vi "ArmExecute.vi"   [LabVIEW 2020]
doc: "Execute Arm VI's\nInputs:\n\nOutputs:"
uses:
  ArmGamePiecePreset.ctl
  <vilib>/Rock Robotics/WPI/ThirdParty/JAS_Junk/TrajLib/Timer_New.vi
  ArmGlobal.vi
  <vilib>/Utility/semaphor.llb/Obtain Semaphore Reference.vi
  <vilib>/Rock Robotics/WPI/ThirdParty/JAS_Junk/TrajLib/Timer_Reset.vi
  <vilib>/Rock Robotics/WPI/ThirdParty/JAS_Junk/TrajLib/Timer_Start.vi
  <vilib>/Rock Robotics/WPI/ThirdParty/JAS_Junk/TrajLib/Timer_HasPeriodPassedOnce.vi
  <vilib>/Rock Robotics/Network Tables/NT Write Boolean.vi
  <vilib>/Rock Robotics/WPI/ThirdParty/JAS_Junk/TrajLib/Trajectory_Library.lvlib
  <vilib>/Rock Robotics/WPI/ThirdParty/PhotonVisionLib/PhotonVisionLib.lvlib
types:
  T1 = typedef "ArmGamePiecePreset.ctl" = enum16{"Cube", "Cone"}
  T2 = typedef "WPI_MotorControlDeviceRef.ctl" = cluster{"DeviceStatus":errorcluster, "Type":T3, "PWM":cluster{"PWM Channel":T4, "DeadBand":T5}, "CAN":cluster{"Device Number":u8, "SetOutput VI Ref":variant, "GetOutput VI Ref":variant, "Enable VI Ref":variant, "Disable VI Ref":variant, "Data":variant}, "Invert":bool, "DIO PWM":cluster{"PWM \"Enable\" Channel":T4, "DIOChannel":T6, "PWM Rate":dbl}}
  T3 = typedef "WPI_MotorControlType.ctl" = enum16{"PWM", "CAN", "DIO PWM"}
  T4 = typedef "FPGA_DIOPWMChannel.ctl" = enum8{"PWM 0", "PWM 1", "PWM 2", "PWM 3", "PWM 4", "PWM 5", "PWM 6", "PWM 7", "PWM 8", "PWM 9", "PWM MXP 0", "PWM MXP 1", "PWM MXP 2", "PWM MXP 3", "PWM MXP 4", "PWM MXP 5", "PWM MXP 6", "PWM MXP 7", "PWM MXP 8", "PWM MXP 9", "Invalid"}
  T5 = typedef "WPI_PWMDeadband.ctl" = cluster{"Name":string, "maxPositivePwm":i32, "minPositivePwm":i32, "centerPwm":i32, "maxNegativePwm":i32, "minNegativePwm":i32, "angularRange":u16}
  T6 = typedef "FPGA_DIOChannel.ctl" = enum8{"DIO 0", "DIO 1", "DIO 2", "DIO 3", "DIO 4", "DIO 5", "DIO 6", "DIO 7", "DIO 8", "DIO 9", "DIO MXP 0", "DIO MXP 1", "DIO MXP 2", "DIO MXP 3", "DIO MXP 4", "DIO MXP 5", "DIO MXP 6", "DIO MXP 7", "DIO MXP 8", "DIO MXP 9", "DIO MXP 10", "DIO MXP 11", "DIO MXP 12", "DIO MXP 13", "DIO MXP 14", "DIO MXP 15", "SPI Port CS1", "SPI Port CS2", "SPI Port CS3", "SPI Port MISO", "SPI Port MOSI", "Invalid"}
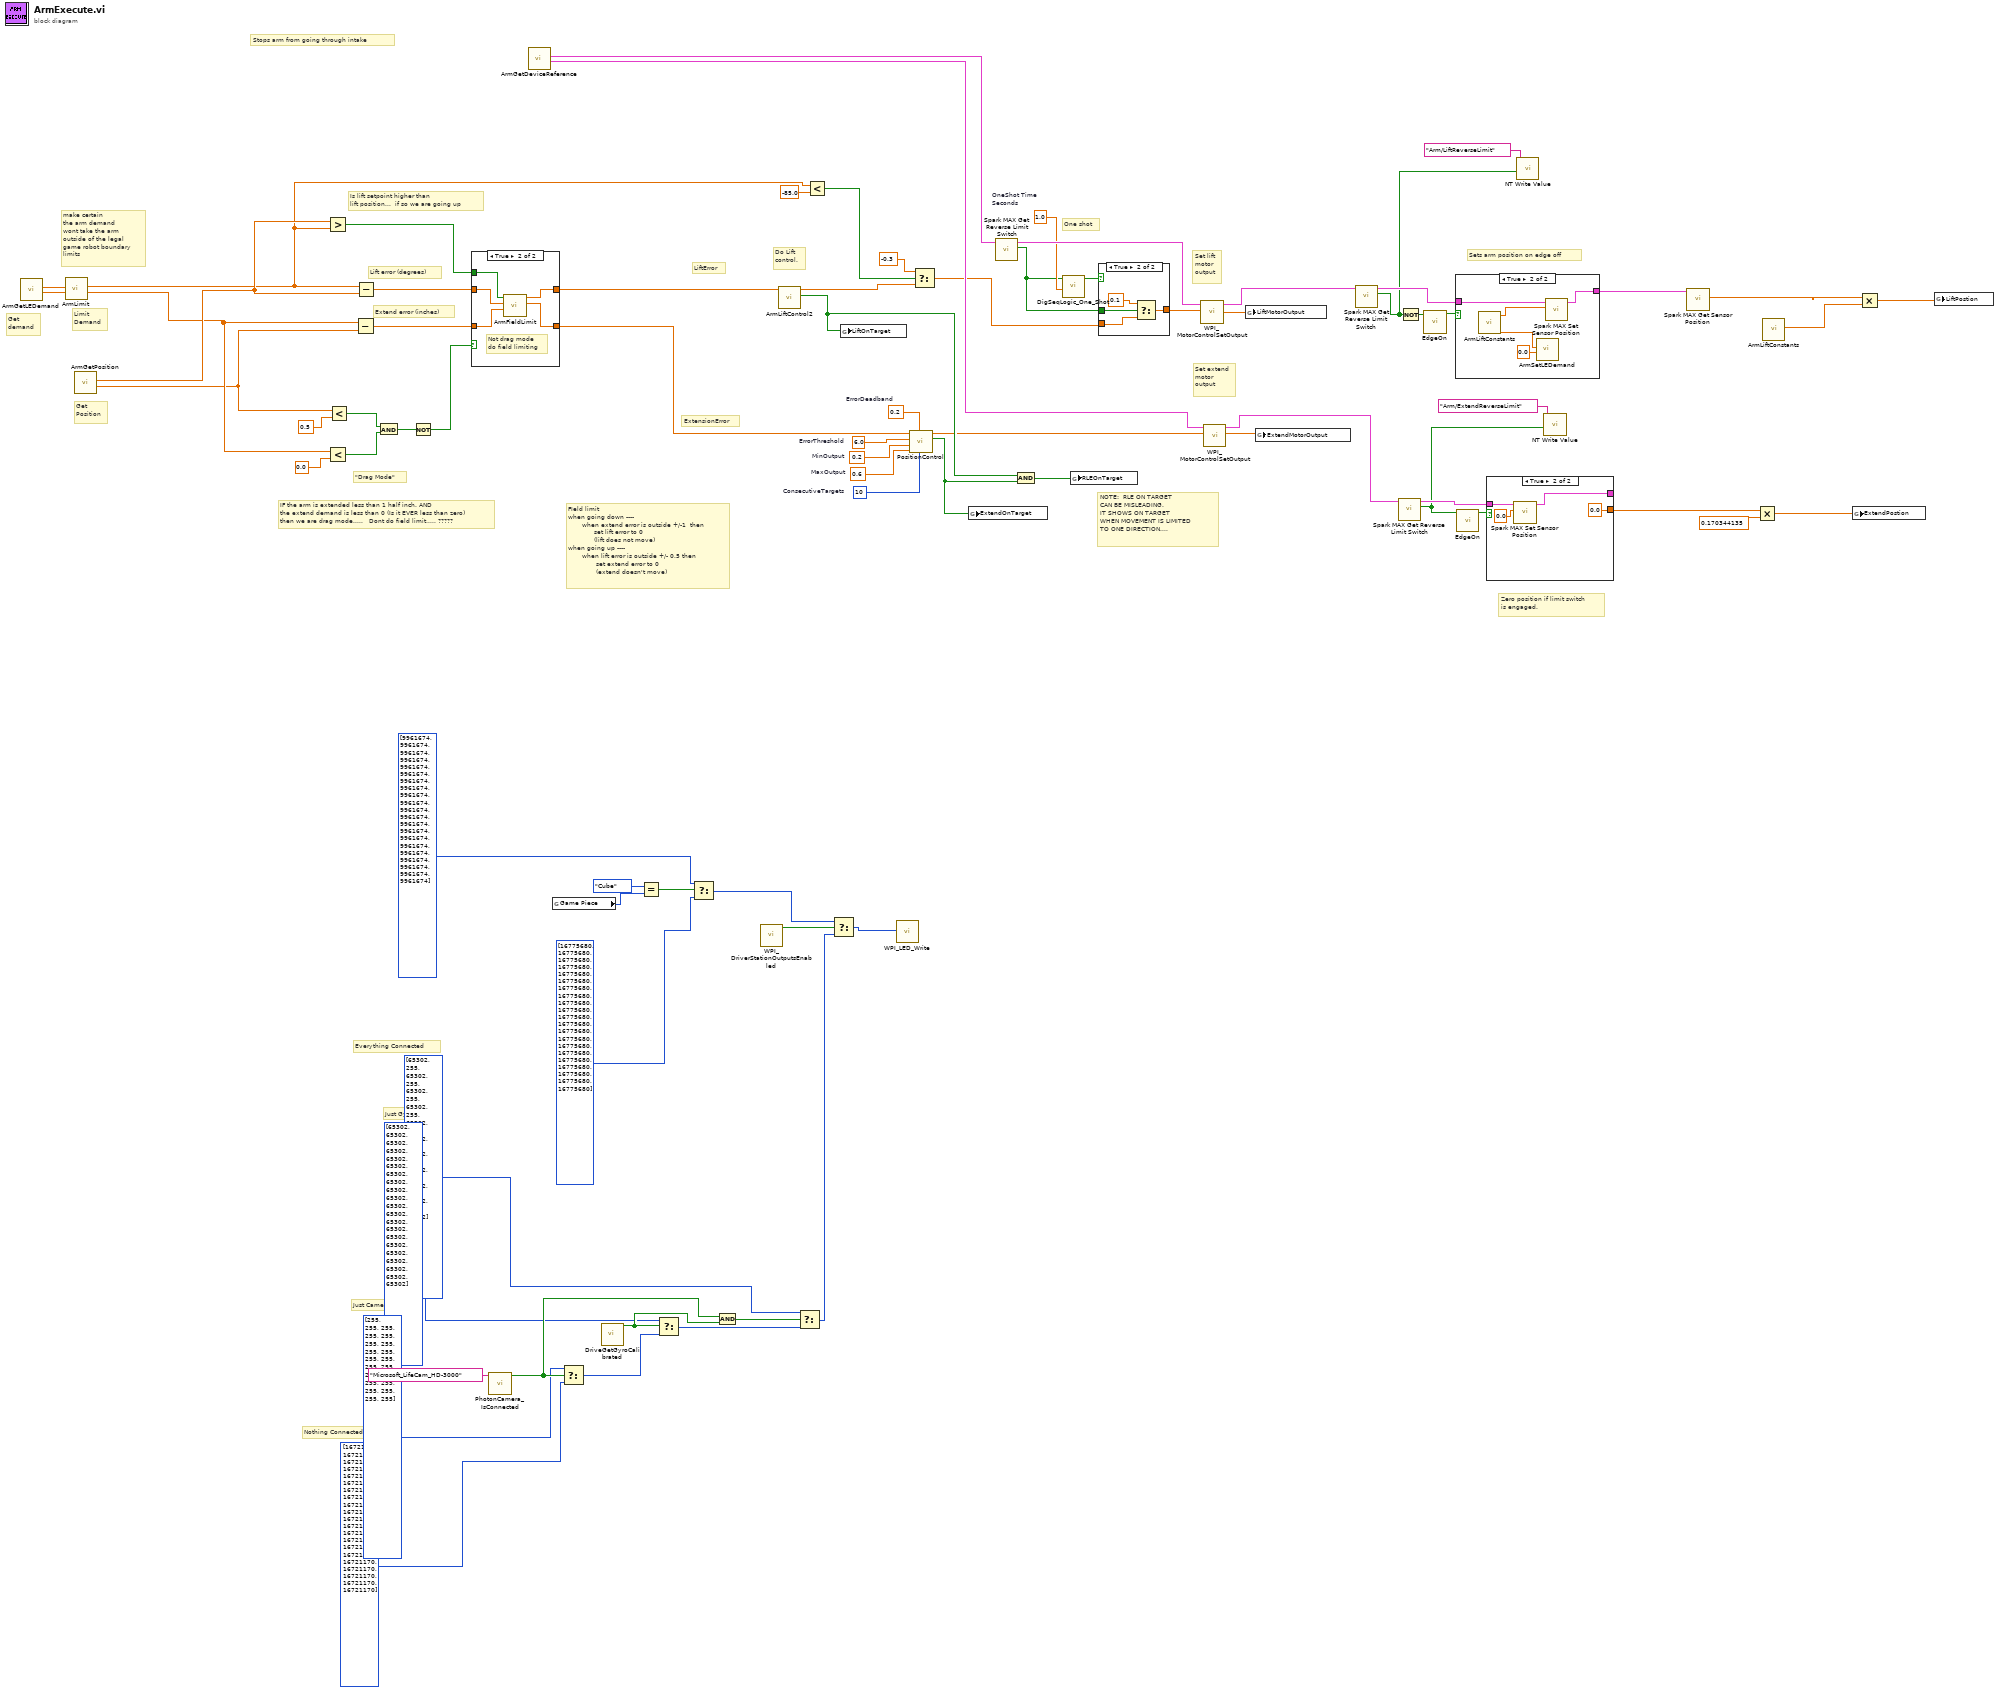
[diagram p0: block diagram]
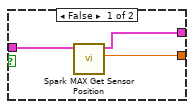
[diagram p5: hidden frame]
diagram:
  w25 = 1.0  # OneShot Time Seconds
  w70 = 10  # ConsecutiveTargets
  w71 = 0.6  # MaxOutput
  w72 = 0.2  # MinOutput
  w73 = 6.0  # ErrorThreshold
  w74 = 0.2  # ErrorDeadband
  # "Zero position if limit switch\nis engaged."
  # "Set extend\nmotor\noutput"
  # "Set lift\nmotor\noutput"
  # "Do Lift\ncontrol."
  # "Extend error (inches)"
  # "Lift error (degrees)"
  # "NOTE:  RLE ON TARGET\nCAN BE MISLEADING.\nIT SHOWS ON TARGET\nWHEN MOVEMENT IS LIMITED \nTO ONE DIRECTION...."
  # "Get\nPosition"
  # "Limit\nDemand"
  # "Get\ndemand"
  # "make certain\nthe arm demand\nwont take the arm\noutside of the legal\ngame robot boundary\nlimits"
  # "FIeld limit\nwhen going down ----\n       when extend error is outside +/-1  then\n             set lift error to 0\n             (lift does not move)\nwhen going up ----\n       when lift error is outside +/- 0.5 then\n              set extend error to 0\n              (extend doesn't move)"
  # "IF the arm is extended less than 1 half inch. AND\nthe extend demand is less than 0 (Is it EVER less than zero)\nthen we are drag mode.....   Dont do field limit..... ?????"
  # "Is lift setpoint higher than\nlift position...  if so we are going up"
  # "Everything Connected"
  # "Just Gyro"
  # "Just Camera"
  # "Nothing Connected"
  # "One shot"
  # "Sets arm position on edge off"
  # "\"Drag Mode\""
  # "Stops arm from going through intake"
  # "ExtensionError"
  # "LiftError"
  n1 = call "ArmGetLEDemand.vi"() -> ("ExtendPositonDemand(in)"=w62:dbl, "LiftPositionDemand(d)"=w63:dbl)  [unwired: 10 in]
  n2 = call "ArmLimit.vi"("Extend"=w62, "Lift"=w63) -> ("Extend"=w31:dbl, "Lift"=w38:dbl)  [unwired: 8 in]
  n3 = call "ArmGetPosition.vi"() -> ("ExtendPostion"=w28:dbl, "LiftPostion"=w51:dbl)  [unwired: 10 in]
  n4 = Greater?(x=w51, y=w38) -> (0:w54:bool)
  n5 = Less?(x=w31, y=0.0) -> (x < y?=w29:bool)
  n6 = Less?(x=w28, y=0.5) -> (x < y?=w30:bool)
  n7 = Subtract(x=w31, y=w28) -> (x-y=w55:dbl)
  n8 = Subtract(x=w38, y=w51) -> (x-y=w50:dbl)
  n9 = And(x=w30, y=w29) -> (x .and. y?=w26:bool)
  n10 = Not(x=w26) -> (.not. x?=w22:bool)
  n11 = case shown="True" w22 {
    tunnel: w55 -> [w78 w84]
    tunnel: w50 -> [w79 w83]
    tunnel: w54 -> [_ w82]
    tunnel: [w79 w81] -> w53
    tunnel: [w78 w80] -> w52
    frame False {
    }
    frame True {
      # "Not drag mode\ndo field limiting"
      n12 = call "ArmFieldLimit.vi"("Extend Error"=w84, "Lift Error"=w83, "Going Down?"=w82) -> ("Extend Error"=w80:dbl, "Lift Error"=w81:dbl)  [unwired: 7 in]
    }
  }
  n13 = call <vilib>:"PhotonCamera_IsConnected.vi"("CameraName"="Microsoft_LifeCam_HD-3000") -> ("IsConnected"=w6:bool)  [unwired: 9 in, 1 out]
  n14 = call "ArmGetDeviceReference.vi"() -> ("armExtend"=w77:T2, "armLift"=w42:T2)  [unwired: 10 in]
  n15 = global read "ArmGlobal.vi" "Game Piece"() -> (w21:T1)
  n16 = Select(t=u32[] [255, 255, 255, 255, 255, 255, 255, 255, 255, 255, 255, 255, 255, 255, 255, 255, 255, 255, 255, 255, 255] ("Color Array"), s=w6, f=u32[] [16721170, 16721170, 16721170, 16721170, 16721170, 16721170, 16721170, 16721170, 16721170, 16721170, 16721170, 16721170, 16721170, 16721170, 16721170, 16721170, 16721170, 16721170, 16721170, 16721170, 16721170] ("Color Array")) -> (s? t:f=w11:u32[])
  n17 = call "DriveGetGyroCalibrated.vi"() -> ("GryoCalibrated"=w7:bool)  [unwired: 11 in]
  n18 = Equal?(x=ArmGamePiecePreset."Cube", y=w21) -> (x = y?=w19:bool)
  n19 = Select(t=u32[] [65302, 65302, 65302, 65302, 65302, 65302, 65302, 65302, 65302, 65302, 65302, 65302, 65302, 65302, 65302, 65302, 65302, 65302, 65302, 65302, 65302] ("Color Array"), s=w7, f=w11) -> (s? t:f=w9:u32[])
  n20 = Select(t=u32[] [9961674, 9961674, 9961674, 9961674, 9961674, 9961674, 9961674, 9961674, 9961674, 9961674, 9961674, 9961674, 9961674, 9961674, 9961674, 9961674, 9961674, 9961674, 9961674, 9961674, 9961674] ("Color Array"), s=w19, f=u32[] [16775680, 16775680, 16775680, 16775680, 16775680, 16775680, 16775680, 16775680, 16775680, 16775680, 16775680, 16775680, 16775680, 16775680, 16775680, 16775680, 16775680, 16775680, 16775680, 16775680, 16775680] ("Color Array")) -> (s? t:f=w15:u32[])
  n21 = And(x=w6, y=w7) -> (x .and. y?=w8:bool)
  n22 = call <vilib>:"WPI_DriverStationOutputsEnabled.vi"() -> ("OutputsEnabled?"=w14:bool)  [unwired: 10 in, 1 out]
  n23 = call "ArmLiftControl2.vi"("erronIn(d)"=w53) -> ("OnTarget"=w56:bool, "motorOutput"=w35:dbl)  [unwired: 9 in]
  n24 = Select(t=u32[] [65302, 255, 65302, 255, 65302, 255, 65302, 255, 65302, 255, 65302, 255, 65302, 255, 65302, 255, 65302, 255, 65302, 255, 65302] ("Color Array"), s=w8, f=w9) -> (s? t:f=w13:u32[])
  n25 = Less?(x=w38, y=-85.0) -> (x < y?=w37:bool)
  n26 = Select(t=w15, s=w14, f=w13) -> (s? t:f=w16:u32[])
  n27 = global write "ArmGlobal.vi" "LiftOnTarget"(w56) -> ()
  n28 = call <vilib>:"WPI_LED_Write.vi"("Color Array"=w16) -> ()  [unwired: 10 in, 1 out]
  n29 = call "PositionControl.vi"("ConsecutiveTargets"=w70, "ErrorDeadband"=w74, "MaxOutput"=w71, "MinOutput"=w72, "ErrorThreshold"=w73, "Error"=w52) -> ("OnTarget"=w69:bool, "OutputValue"=w45:dbl)  [unwired: 3 in, 1 out]
  n30 = Select(t=-0.3, s=w37, f=w35) -> (s? t:f=w36:dbl)
  n31 = global write "ArmGlobal.vi" "ExtendOnTarget"(w69) -> ()
  n32 = call <vilib>:"Spark MAX Get Reverse Limit Switch.vi"("MotorControlDevRef in"=w42) -> ("Hard Limit Rev"=w24:bool, "MotorControlDevRef out"=w43:T2)  [unwired: 7 in, 2 out]
  n33 = And(x=w56, y=w69) -> (x .and. y?=w68:bool)
  n34 = call <vilib>:"DigSeqLogic_One_Shot.vi"("OneShot"=w25, "Input"=w24) -> ("Output"=w23:bool)  [unwired: 8 in, 1 out]
  n35 = global write "ArmGlobal.vi" "RLEOnTarget"(w68) -> ()
  n36 = case shown="True" w23 {
    tunnel: [w85 w89] -> w58
    tunnel: w36 -> [w85 w87]
    tunnel: w24 -> [_ w86]
    frame False {
    }
    frame True {
      n37 = Select(t=0.1, s=w86, f=w87) -> (s? t:f=w89:dbl)
    }
  }
  n38 = call <vilib>:"WPI_MotorControlSetOutput.vi"("Output"=w58, "MotorControlDevRef"=w43) -> ("Motor Output"=w75:dbl, "MotorControlDevRef"=w44:T2)  [unwired: 7 in, 1 out]
  n39 = call <vilib>:"WPI_MotorControlSetOutput.vi"("Output"=w45, "MotorControlDevRef"=w77) -> ("Motor Output"=w76:dbl, "MotorControlDevRef"=w64:T2)  [unwired: 7 in, 1 out]
  n40 = global write "ArmGlobal.vi" "LiftMotorOutput"(w75) -> ()
  n41 = global write "ArmGlobal.vi" "ExtendMotorOutput"(w76) -> ()
  n42 = call <vilib>:"Spark MAX Get Reverse Limit Switch.vi"("MotorControlDevRef in"=w44) -> ("Hard Limit Rev"=w40:bool, "MotorControlDevRef out"=w48:T2)  [unwired: 7 in, 2 out]
  n43 = call <vilib>:"Spark MAX Get Reverse Limit Switch.vi"("MotorControlDevRef in"=w64) -> ("Hard Limit Rev"=w1:bool, "MotorControlDevRef out"=w60:T2)  [unwired: 7 in, 2 out]
  n44 = Not(x=w40) -> (.not. x?=w46:bool)
  n45 = call "EdgeOn.vi"("Current State"=w46) -> ("Edge On Found"=w47:bool)  [unwired: 10 in]
  n46 = case shown="True" w47 {
    tunnel: w48 -> [w90 w95]
    tunnel: [w90 w94] -> w49
    frame False {
    }
    frame True {
      n47 = call "ArmLiftConstants.vi"() -> ("Starting Angle"=w91:dbl, "StartingArmPos"=w93:dbl)  [unwired: 8 in, 2 out]
      n48 = call "ArmSetLEDemand.vi"("SetExtendPositonDemand(in)"=0.0, "SetLIftPostionDemand(d)"=w91) -> ()  [unwired: 9 in, 1 out]
      n49 = call <vilib>:"Spark MAX Set Sensor Position.vi"("Position"=w93, "MotorControlDeviceRef"=w95) -> ("MotorControlDeviceRef"=w94:T2)  [unwired: 8 in, 1 out]
    }
  }
  n50 = call "EdgeOn.vi"("Current State"=w1) -> ("Edge On Found"=w59:bool)  [unwired: 10 in]
  n51 = case shown="True" w59 {
    tunnel: w60 -> [w98 w102]
    tunnel: [w97 w101] -> _
    tunnel: [w96 0.0 ("Sensor Position")] -> w33
    frame False {
      n52 = call <vilib>:"Spark MAX Get Sensor Position.vi"("MotorControlDevRef in"=w98) -> ("Sensor Position"=w96:dbl, "MotorControlDevRef out"=w97:T2)  [unwired: 7 in, 2 out]
    }
    frame True {
      n53 = call <vilib>:"Spark MAX Set Sensor Position.vi"("Position"=0.0, "MotorControlDeviceRef"=w102) -> ("MotorControlDeviceRef"=w101:T2)  [unwired: 8 in, 1 out]
    }
  }
  n54 = call-poly <vilib>:"NT Write Value.vi"("value"=w40, "name"="Arm/LiftReverseLimit") -> ()  [unwired: 9 in, 1 out]
  n55 = call-poly <vilib>:"NT Write Value.vi"("value"=w1, "name"="Arm/ExtendReverseLimit") -> ()  [unwired: 9 in, 1 out]
  n56 = call <vilib>:"Spark MAX Get Sensor Position.vi"("MotorControlDevRef in"=w49) -> ("Sensor Position"=w65:dbl)  [unwired: 7 in, 3 out]
  n57 = Multiply(x=w33, y=0.170344135) -> (x*y=w61:dbl)
  n58 = call "ArmLiftConstants.vi"() -> ("LiftConversionFactor"=w57:dbl)  [unwired: 8 in, 3 out]
  n59 = global write "ArmGlobal.vi" "ExtendPostion"(w61) -> ()
  n60 = Multiply(x=w65, y=w57) -> (x*y=w67:dbl)
  n61 = global write "ArmGlobal.vi" "LiftPostion"(w67) -> ()
